vi "UDP Comm Dev.vi"() -> ()   [LabVIEW 2009]
uses:
  Remote Control/Message Type.ctl
  <vilib>/Platform/TimedLoop/XDataNode/XDataNode.xnode
  <vilib>/Platform/TimedLoop/XDataNode/nitl_modes.ctl
  <vilib>/Platform/TimedLoop/XDataNode/XDNodeRunTimeDep.lvlib
  <vilib>/Platform/TimedLoop/XDataNode/wakeup.ctl
  <vilib>/Platform/TimedLoop/XDataNode/timing_clust.ctl
  <vilib>/Platform/TimedLoop/XDataNode/loadlvalarms.vi
  Remote Control/Motor Command.ctl
  Remote Control/Control Message.ctl
panel:
  in  "Read Timeout":i32=1000
  in  "Local Port":u16=8800
  in  "Control Message":T1
  out "YOUNG CHANGEME\nroute this to whereever\nmotor commands go":T2
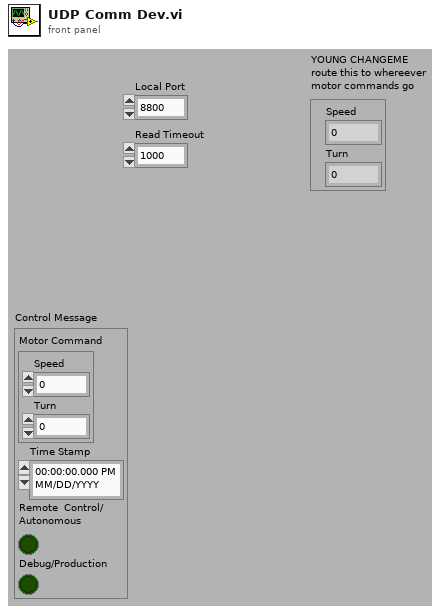
[diagram p1: front panel]
types:
  T1 = typedef "Control Message.ctl" = cluster{"Motor Command":T2, "Time Stamp":timestamp, "Remote  Control/\nAutonomous":bool, "Debug/Production":bool}
  T2 = typedef "Motor Command.ctl" = cluster{"Speed":i16, "Turn":i16}
  T3 = typedef "XDNodeRunTimeDep.lvlib/timing_clust.ctl" = cluster{"Expected End [f-1]":u64, "Actual End [f-1]":u64, "Finished Late? [f-1]":bool, "Expected End [i-1]":u64, "Actual End [i-1]":u64, "Finished Late? [i-1]":bool, "Expected Start [i]":u64, "Actual Start [i]":u64, "Expected Start [f]":u64, "Actual Start [f]":u64, "Source Name":string, "Structure Name":string, "Period":i64, "Deadline":i64, "Offset":i64, "Start":i64, "Priority":i32, "Timeout":i32, "Mode":T4, "Wakeup Reason":T5, "Error":errorcluster, "Source Type":string, "Secondary Source Type":string, "Global End Time":u64, "Global Start Time":u64, "Frame Duration":u64, "Iteration Duration":u64, "Assigned CPU":i32, "I/O Scan Engine Mode":u32}
  T4 = typedef "XDNodeRunTimeDep.lvlib/nitl_modes.ctl" = enum32{"No Change", "Process missed periods, maintain original phase", "Discard missed periods, maintain original phase", "Process missed periods, ignore original phase", "Discard missed periods, ignore original phase"}
  T5 = typedef "XDNodeRunTimeDep.lvlib/wakeup.ctl" = enum32{"Normal", "Aborted", "Asynchronous wakeup", "Timing source error", "Timed loop error", "Timeout"}
  T6 = typedef "UDP Base.ctl" = cluster{"UDP Session":refnum<k16>, "UDP Socket Params":T7}
  T7 = typedef "UDP Socket Params.ctl" = cluster{"Local Port":u16, "Read Timeout":i32, "Write Timeout":i32}
  T8 = typedef "Message Type.ctl" = enum16{"Motor Command", "Debug Data"}
  T9 = typedef "UDP Network Location.ctl" = cluster{"IP Address":string, "Port":u16}
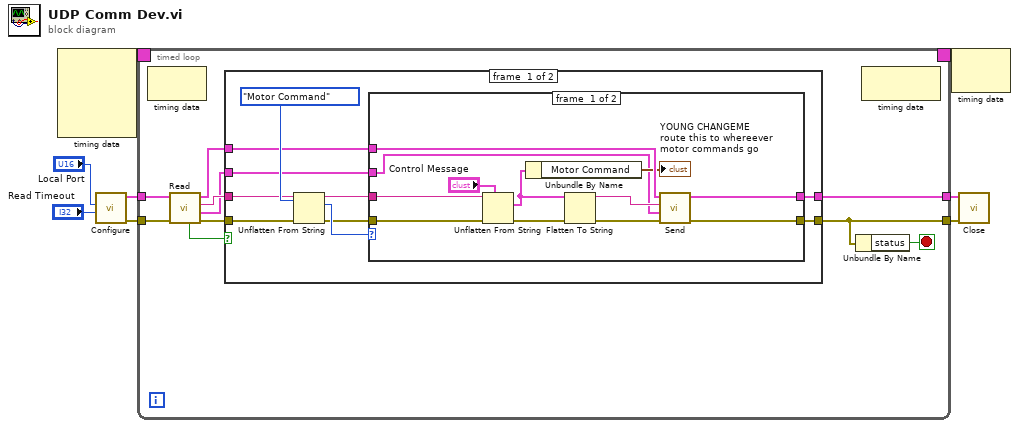
[diagram p0: block diagram]
diagram:
  n1 = node-c288() -> (w2:T3)  [unwired: 4 in]
  n2 = call "Configure.vi"("Read Timeout"="Read Timeout", "Local Port"="Local Port") -> ("error out"=w7:errorcluster, "UDP Base out"=w8:T6)  [unwired: 8 in]
  n3 = timed-loop {
    tunnel: w8 -> [w16]
    tunnel: w7 -> [w15]
    tunnel: [w18] -> w5
    tunnel: [w17] -> w6
    timing: w2 -> [_]
    timing-out: [_] -> w1
    stop <- w9 stop-if-true
    n4 = node-c288() -> ()  [unwired: 1 in, 1 out]
    n5 = call "Read.vi"("error in (no error)"=w15, "UDP Base in"=w16) -> ("error out"=w13:errorcluster, "Network Location"=w10:T9, "Receive Data"=w12:string, "UDP Base out"=w14:T6, "Timeout"=w11:bool)  [unwired: 4 in, 1 out]
    n6 = case shown="False" w11 {
      tunnel: [w28 w45] -> w18
      tunnel: [w27 w46] -> w17
      tunnel: w14 -> [w24 w46]
      tunnel: w13 -> [w23 w45]
      tunnel: w12 -> [w22 _]
      tunnel: w10 -> [w21 _]
      frame #0 {
        n7 = Unflatten From String(type=Message_Type."Motor Command" ("Message Type"), binary string=w22, error in (no error)=w23) -> (rest of the binary string=w25:string, value=w29:T8, error out=w26:errorcluster)  [unwired: 2 in]
        n8 = case shown="\"Motor Command\", Default" w29 {
          tunnel: [w36 w44] -> w28
          tunnel: [w37 w43] -> w27
          tunnel: w26 -> [w42 w44]
          tunnel: w25 -> [w41 _]
          tunnel: w24 -> [w34 w43]
          tunnel: w21 -> [w31 _]
          frame #0 {
            n9 = Unflatten From String(type="Control Message", binary string=w41, error in (no error)=w42) -> (value=w33:T1, error out=w40:errorcluster)  [unwired: 2 in, 1 out]
            n10 = Unbundle By Name(w33) -> ("Motor Command"=→"YOUNG CHANGEME\nroute this to whereever\nmotor commands go":T2)
            n11 = Flatten To String(anything=w33, error in (no error)=w40) -> (data string=w35:string, error out=w38:errorcluster)  [unwired: 2 in, 1 out]
            n12 = call "Send.vi"("error in (no error)"=w38, "Destination Location"=w31, "Send Data"=w35, "UDP Base in"=w34) -> ("error out"=w36:errorcluster, "UDP Base out"=w37:T6)  [unwired: 5 in, 1 out]
          }
          frame #1 {
          }
        }
      }
      frame #1 {
      }
    }
    n13 = Unbundle By Name(w18) -> ("status"=w9:bool)
    n14 = node-c288() -> ()  [unwired: 1 in, 1 out]
  }
  n15 = node-c288(w1) -> ()  [unwired: 1 out]
  n16 = call "Close.vi"("error in (no error)"=w5, "Cluster of class private data"=w6) -> ()  [unwired: 9 in, 1 out]
